vi "Bundle.vi"(8 "error in (no error)":errorcluster, 9 "Override data":T1[](array[typedef]), 10 "Iteration Target":i32, 11 "Loop Msg in":refnum<class "Loop Msg.lvclass">) -> (0 "error out":errorcluster, 3 "Loop Msg out":refnum<class "Loop Msg.lvclass">)   [LabVIEW 2020, in "Sequencer.lvlib" / "Loop Msg.lvclass"]
doc: "Write Iteration Target and Overwrite data to the Loop Msg private data. Also set Iteration to 0."
uses:
  Loop Msg.lvclass
  Sequence Editor/Controls/Ctl_FlexDataElements.ctl
  Sequence Editor/Controls/Ctl_FlexDataElement.ctl
  Loop Msg.lvclass/Loop Msg.ctl
  Sequencer.lvlib
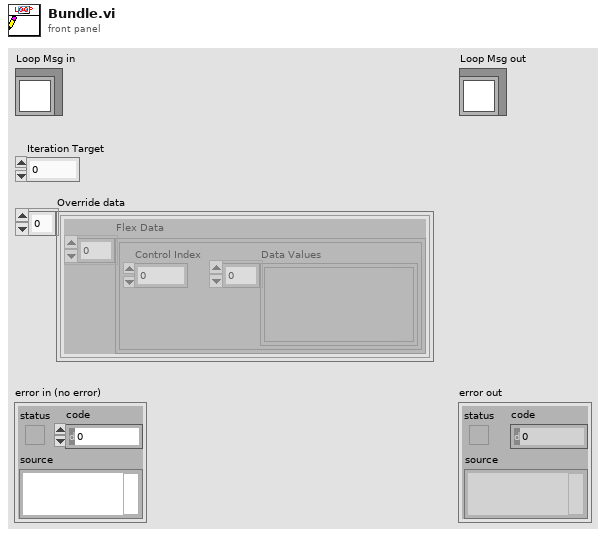
[diagram p1: front panel]
types:
  T1 = typedef "Sequencer.lvlib/Ctl_FlexDataElements.ctl" = cluster{"Flex Data":T2[]}
  T2 = typedef "Sequencer.lvlib/Ctl_FlexDataElement.ctl" = cluster{"Control Index":i32, "Data Values":variant[]}
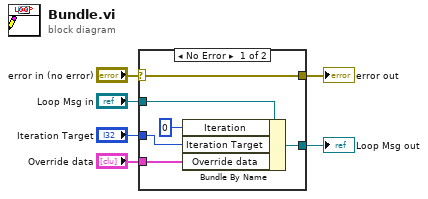
[diagram p0: block diagram]
diagram:
  n1 = case shown="No Error" "error in (no error)" {
    selector: "error in (no error)" -> [w12 w13]
    tunnel: [w12 w13] -> w5
    tunnel: [w10 w14] -> w3
    tunnel: "Loop Msg in" -> [w11 w14]
    tunnel: "Iteration Target" -> [w9 _]
    tunnel: "Override data" -> [w7 _]
    frame No Error {
      n2 = Bundle By Name(cluster=w11, "Iteration"=0, "Iteration Target"=w9, "Override data"=w7) -> (w10:refnum<class "Loop Msg.lvclass">)
    }
    frame Error {
    }
  }
  "error out" <- w5
  "Loop Msg out" <- w3
